vi "ROI entry-Set display mapping.vi"(8 "error in (no error)":errorcluster) -> (0 "error out":errorcluster)   [LabVIEW 2017]
uses:
  ROI Entry screen/Globals/gl_ROI Entry UI globals.vi
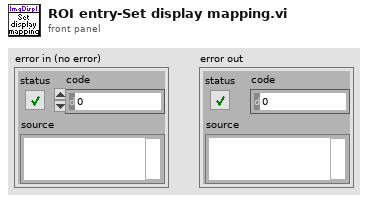
[diagram p1: front panel]
types:
  T1 = cluster{"Conversion Method":u32, "Minimum Value":i32, "Maximum Value":i32, "Number Of Shifts":i32}
  T2 = typedef "ROI entry screen ctrl refs cluster.ctl" = cluster{"Done button":refnum<vi>, "Imaging button":refnum<vi>, "Acquisition button":refnum<vi>, "POI dwell time (us)":refnum<vi>, "Scan dwell time per pixel (us)":refnum<vi>, "# of planes":refnum<vi>, "Zoom Ctrl":refnum<vi>, "Equal size":refnum<vi>, "Channel":refnum<vi>, "Image Display":refnum<vi>, "Z-Plane Selector":refnum<vi>, "Number of lines left":refnum<vi>, "Z-stack folder path":refnum<vi>, "POI Density":refnum<vi>, "Arb Plane Entry":refnum<vi>, "Whole plane":refnum<vi>, "Clear Last":refnum<vi>, "Clear All":refnum<vi>, "Trial Length (sec)":refnum<vi>, "Palette Type":refnum<vi>, "Intensity slider":refnum<vi>, "# POI":refnum<vi>, "Max Z Proj":refnum<vi>, "Zplane ind":refnum<vi>, "Wavelength (nm)":refnum<vi>, "Number of Trials":refnum<vi>, "Funct stim.trig.enable":refnum<vi>, "Funct stim.trig.delay (s)":refnum<vi>, "Line Mode":refnum<vi>, "Step size (µm)":refnum<vi>, "ROI move mode":refnum<vi>, "Cool-down time (s)":refnum<vi>, "Enable cool-down time":refnum<vi>, "Motor Z ind. (um)":refnum<vi>, "AOL Z ind. (um)":refnum<vi>, "Load Reference Image":refnum<vi>}
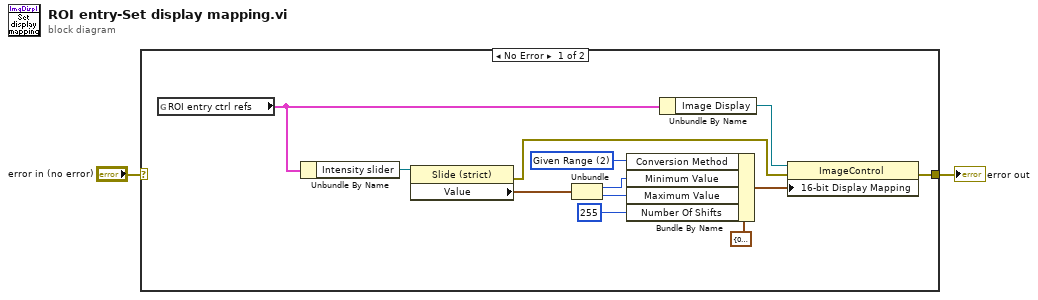
[diagram p0: block diagram]
diagram:
  n1 = case shown="No Error" "error in (no error)" {
    selector: "error in (no error)" -> [_ w15]
    tunnel: [w14 w15] -> w1
    frame No Error {
      w5 = u32 2 items=["Full Dynamic", "Downshift", "Given Range", "90 % Dynamic", "Given Percent Range"] ("Conversion Method")
      n2 = global read "gl_ROI Entry UI globals.vi" "ROI entry ctrl refs"() -> (w11:T2)
      n3 = Unbundle By Name(w11) -> ("Intensity slider"=w9:refnum<vi>)
      n4 = property class="Slide (strict)"(reference=w9) -> (error out=w13:errorcluster, "Value"=w10:cluster{i16, i16})  [unwired: 1 in, 1 out]
      n5 = Unbundle(w10) -> (w3:i16, w4:i16)
      n6 = Bundle By Name(cluster=T1 {"Conversion Method"=0, "Minimum Value"=0, "Maximum Value"=0, "Number Of Shifts"=0} ("16-bit Display Mapping:All Elements"), "Conversion Method"=w5, "Minimum Value"=w3, "Maximum Value"=w4, "Number Of Shifts"=255) -> (w7:T1)
      n7 = Unbundle By Name(w11) -> ("Image Display"=w12:refnum<vi>)
      n8 = property on="Property Node" class="ImageControl"(reference=w12, error in=w13, "16-bit Display Mapping"=w7) -> (error out=w14:errorcluster)  [unwired: 1 out]
    }
    frame Error {
    }
  }
  "error out" <- w1
